vi "ShowCurStep.vi"(8 "error in (no error)":errorcluster, 10 "Step indicator reference":refnum<vi>, 11 "Current step":i32) -> (0 "error out":errorcluster)   [LabVIEW 2017]
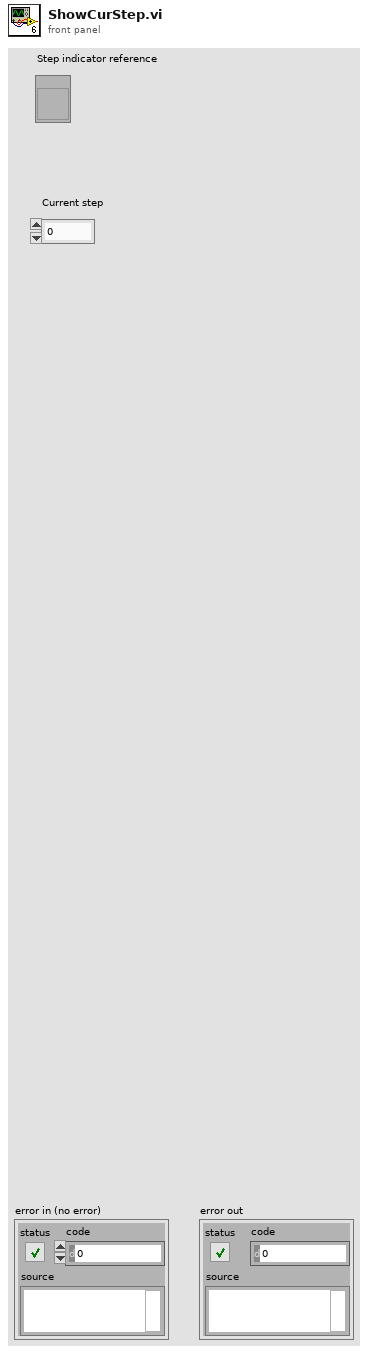
[diagram p1: front panel]
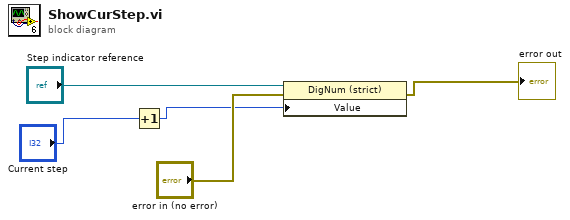
[diagram p0: block diagram]
diagram:
  n1 = Increment(x="Current step") -> (x+1=w1:i32)
  n2 = property class="DigNum (strict)"(reference="Step indicator reference", error in="error in (no error)", "Value"=w1) -> (error out=→"error out":errorcluster)  [unwired: 1 out]
